vi "AutoDetect.vi"(1 "Image":T1) -> (0 "Detection Parameters Out":T2 {"Max Intensity%" max=100 step=1})   [LabVIEW 2013]
uses:
  <vilib>/vision/Image Controls.llb/IMAQ Image.ctl
  <vilib>/vision/NI_Vision_Development_Module.lvlib
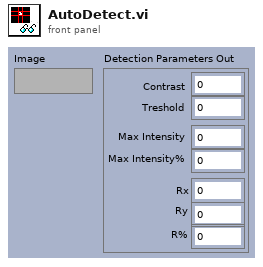
[diagram p1: front panel]
types:
  T1 = typedef "IMAQ Image.ctl" = refnum<image>
  T2 = cluster{"Contrast":i32, "Treshold":u8, "Max Intensity":i32, "Max Intensity%":u8, "Rx":i32, "Ry":i32, "R%":sgl}
  T3 = cluster{"Objects":u16, "Threshold":i32, "Reject Border":bool, "Fill Holes":bool, "Min Object Size":bool, "Min Size":i32, "Max Object Size":bool, "Max Size":i32, "Show Search Area":bool, "Show Center":bool, "Show Bounding Box":bool}
  T4 = typedef "Image Type" = u32
  T5 = cluster{"Object Center":cluster{"X":sgl, "Y":sgl}, "Bounding Box":cluster{"X Left":i32, "Y Top":i32, "X Right":i32, "Y Bottom":i32}, "Area":sgl, "Orientation":sgl, "Aspect Ratio":sgl, "Nb Holes":i32}[]
  T6 = cluster{"Object Center":cluster{"X":sgl, "Y":sgl}, "Bounding Box":cluster{"X Left":i32, "Y Top":i32, "X Right":i32, "Y Bottom":i32}, "Area":sgl, "Orientation":sgl, "Aspect Ratio":sgl, "Nb Holes":i32}
  T7 = cluster{"histogram":u32[], "Minimal Value":sgl, "Maximal Value":sgl, "Starting Value":sgl, "Interval Width":sgl, "Mean Value":sgl, "Standard  Variation":sgl, "Area (pixels)":i32}
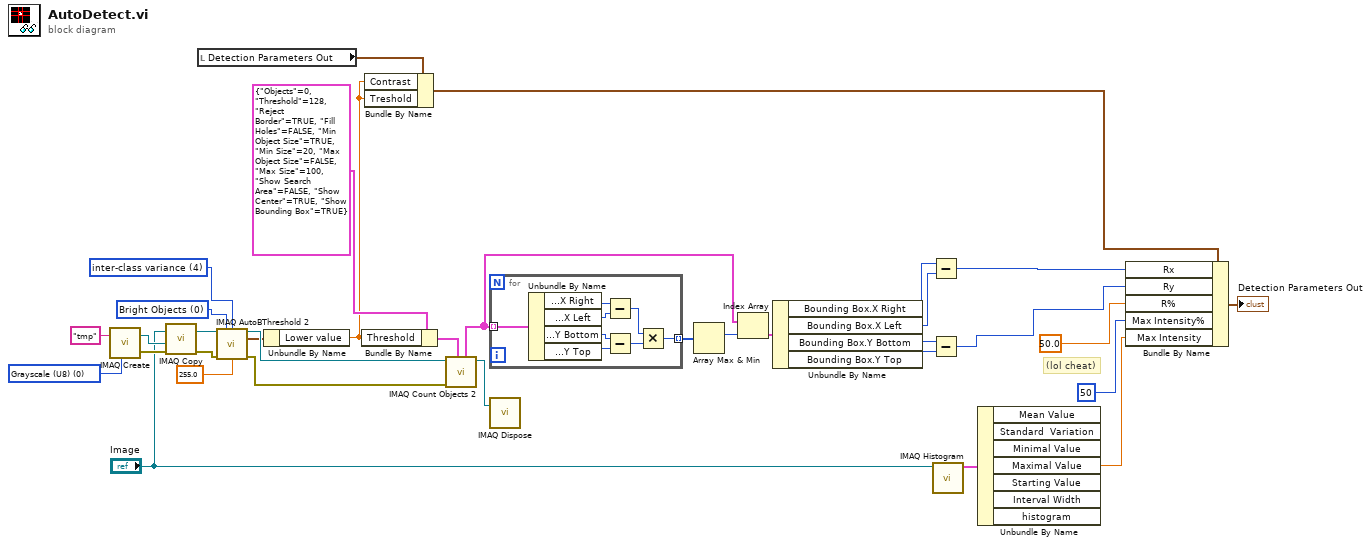
[diagram p0: block diagram]
diagram:
  w12 = 4 items=["clustering", "entropy", "metric", "moments", "inter-class variance"] ("Method (clustering)")
  w13 = u32 0 items=["Bright Objects", "Dark Objects"] ("Look For (Bright Objects)")
  w23 = T4 0 items=["Grayscale (U8)", "Grayscale (I16)", "Grayscale (SGL)", "Complex (CSG)", "RGB (U32)", "HSL (U32)", "RGB (U64)", "Grayscale (U16)"] ("Image Type")
  # "(lol cheat)"
  n1 = call "IMAQ Create"("Image Name"="tmp", "Image Type"=w23) -> ("New Image"=w22:T1, "error out"=w11:errorcluster)  [unwired: 3 in]
  n2 = call "IMAQ Copy"("error in (no error)"=w11, "Image Dst"=w22, "Image Src"="Image") -> ("error out"=w10:errorcluster, "Image Dst Out"=w18:T1)  [unwired: 3 in]
  n3 = local read "Detection Parameters Out"() -> (w21:T2)
  n4 = call "IMAQ AutoBThreshold 2"("Image Src"=w18, "Look For (Bright Objects)"=w13, "Method (clustering)"=w12, "error in (no error)"=w10, "Replace Value (1)"=sgl 255.0) -> ("Image Dst Out"=w17:T1, "Threshold Range Out"=w16:cluster{"Lower value":sgl, "Upper value":sgl}, "error out"=w9:errorcluster)  [unwired: 8 in]
  n5 = Unbundle By Name(w16) -> ("Lower value"=w15:sgl)
  n6 = Bundle By Name(cluster=T3 {"Objects"=0, "Threshold"=128, "Reject Border"=TRUE, "Fill Holes"=FALSE, "Min Object Size"=TRUE, "Min Size"=20, "Max Object Size"=FALSE, "Max Size"=100, "Show Search Area"=FALSE, "Show Center"=TRUE, "Show Bounding Box"=TRUE} ("Settings"), "Threshold"=w15) -> (w31:T3)
  n7 = Bundle By Name(cluster=w21, "Contrast"=w15, "Treshold"=w15) -> (w20:T2)
  n8 = call "IMAQ Count Objects 2"("Settings"=w31, "error in (no error)"=w9, "Image"=w17) -> ("Image Out"=w4:T1, "Objects"=w32:T5)  [unwired: 4 in, 3 out]
  n9 = for {
    tunnel: w32 -> [w42] mode=indexing
    tunnel: [w35] -> w34 mode=indexing
    n10 = Unbundle By Name(w42) -> ("Bounding Box.X Right"=w41:i32, "Bounding Box.X Left"=w40:i32, "Bounding Box.Y Bottom"=w38:i32, "Bounding Box.Y Top"=w39:i32)
    n11 = Subtract(x=w41, y=w40) -> (x-y=w37:i32)
    n12 = Subtract(x=w38, y=w39) -> (x-y=w36:i32)
    n13 = Multiply(x=w37, y=w36) -> (x*y=w35:i32)
  }
  n14 = call "IMAQ Dispose"("Image"=w4) -> ()  [unwired: 5 in, 1 out]
  n15 = Array Max & Min(array=w34) -> (max index (indices)=w33:i32)  [unwired: 3 out]
  n16 = Index Array(array=w32, index=w33) -> (element=w26:T6)
  n17 = Unbundle By Name(w26) -> ("Bounding Box.X Right"=w30:i32, "Bounding Box.X Left"=w29:i32, "Bounding Box.Y Bottom"=w28:i32, "Bounding Box.Y Top"=w27:i32)
  n18 = Subtract(x=w30, y=w29) -> (x-y=w2:i32)
  n19 = Subtract(x=w28, y=w27) -> (x-y=w1:i32)
  n20 = call "IMAQ Histogram"("Image"="Image") -> ("Histogram Report"=w6:T7)  [unwired: 4 in, 6 out]
  n21 = Unbundle By Name(w6) -> ("Maximal Value"=w5:sgl)  [unwired: 6 out]
  n22 = Bundle By Name(cluster=w20, "Rx"=w2, "Ry"=w1, "R%"=50.0 ("y"), "Max Intensity%"=u8 50, "Max Intensity"=w5) -> (→"Detection Parameters Out":T2)
